vi "Timer.vi"(3 "Set Timer":dbl, 5 "Start":bool) -> (0 "Remaining Time":dbl, 1 "End Loop":bool, 2 "Elapsed Time":dbl)   [LabVIEW 2024]
uses:
  Global Varibles.vi
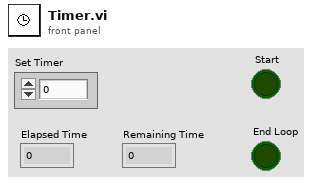
[diagram p1: front panel]
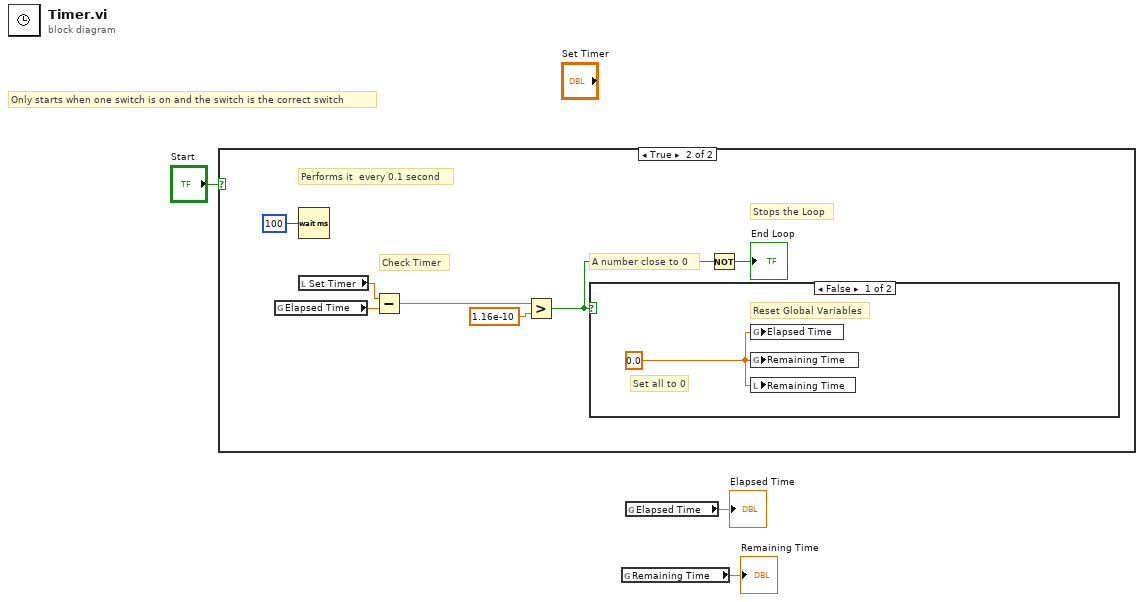
[diagram p0: block diagram]
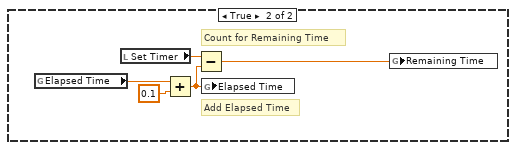
[diagram p3: hidden frame]
diagram:
  # "Only starts when one switch is on and the switch is the correct switch"
  n1 = case shown="True" "Start" {
    frame False {
    }
    frame True {
      # "A number close to 0"
      # "Performs it  every 0.1 second"
      # "Check Timer"
      # "Stops the Loop"
      n2 = global read "Global Varibles.vi" "Elapsed Time"() -> (w7:dbl)
      n3 = Wait (ms)(milliseconds to wait=u32 100) -> ()  [unwired: 1 out]
      n4 = local read "Set Timer"() -> (w9:dbl)
      n5 = Subtract(x=w9, y=w7) -> (x-y=w6:dbl)
      n6 = Greater?(x=w6, y=1.16e-10) -> (0:w5:bool)
      n7 = case shown="False" w5 {
        frame False {
          w11 = 0.0 ("Elapsed Time")
          # "Set all to 0"
          # "Reset Global Variables"
          n8 = global write "Global Varibles.vi" "Elapsed Time"(w11) -> ()
          n9 = global write "Global Varibles.vi" "Remaining Time"(w11) -> ()
          n10 = local write "Remaining Time"(w11) -> ()
        }
        frame True {
          # "Count for Remaining Time"
          # "Add Elapsed Time"
          n11 = global read "Global Varibles.vi" "Elapsed Time"() -> (w15:dbl)
          n12 = local read "Set Timer"() -> (w16:dbl)
          n13 = Add(x=w15, y=0.1) -> (x+y=w14:dbl)
          n14 = Subtract(x=w16, y=w14) -> (x-y=w13:dbl)
          n15 = global write "Global Varibles.vi" "Elapsed Time"(w14) -> ()
          n16 = global write "Global Varibles.vi" "Remaining Time"(w13) -> ()
        }
      }
      n17 = Not(x=w5) -> (.not. x?=→"End Loop":bool)
    }
  }
  n18 = global read "Global Varibles.vi" "Remaining Time"() -> (→"Remaining Time":dbl)
  n19 = global read "Global Varibles.vi" "Elapsed Time"() -> (→"Elapsed Time":dbl)
